vi "Read Configuration Data.vi"(8 "error in":errorcluster) -> (0 "error out":errorcluster, 3 "Configuration Data":T1)   [LabVIEW 2014]
uses:
  Configuration Data.ctl
  controls/MHL Configuration.ctl
  Controller/Controller Configuration.ctl
  Boiler/Boiler Configuration.ctl
  Boiler System Globals.vi
  <vilib>/Utility/config.llb/NI_LVConfig.lvlib
  Controller/Controller.lvlib
  Boiler/Boiler.lvlib
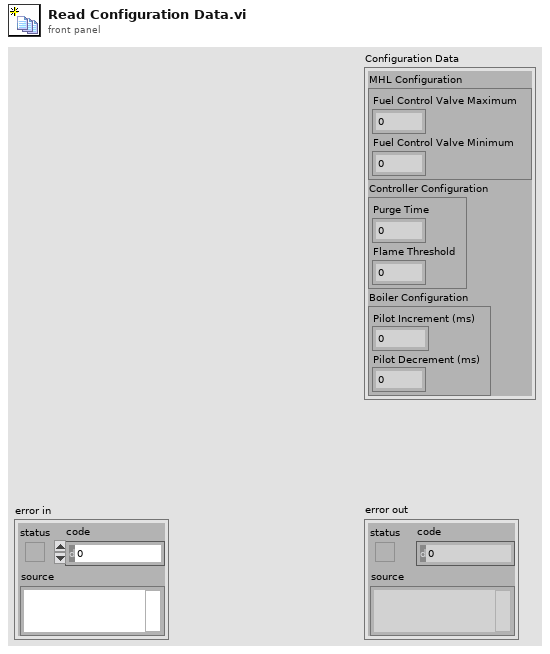
[diagram p1: front panel]
types:
  T1 = typedef "Configuration Data.ctl" = cluster{"MHL Configuration":T2, "Controller Configuration":T3, "Boiler Configuration":T4}
  T2 = typedef "MHL Configuration.ctl" = cluster{"Fuel Control Valve Maximum":dbl, "Fuel Control Valve Minimum":dbl}
  T3 = typedef "Controller.lvlib/Controller Configuration.ctl" = cluster{"Purge Time":u32, "Flame Threshold":u32}
  T4 = typedef "Boiler.lvlib/Boiler Configuration.ctl" = cluster{"Pilot Increment (ms)":u32, "Pilot Decrement (ms)":u32}
  T5 = enum32{"invalid app kind", "Development System", "Run Time System", "Student Edition", "Embedded LabVIEW", "Evaluation", "Custom"}
  T6 = typedef "NI_LVConfig.lvlib/Config Data RefNum.ctl" = refnum<k1>
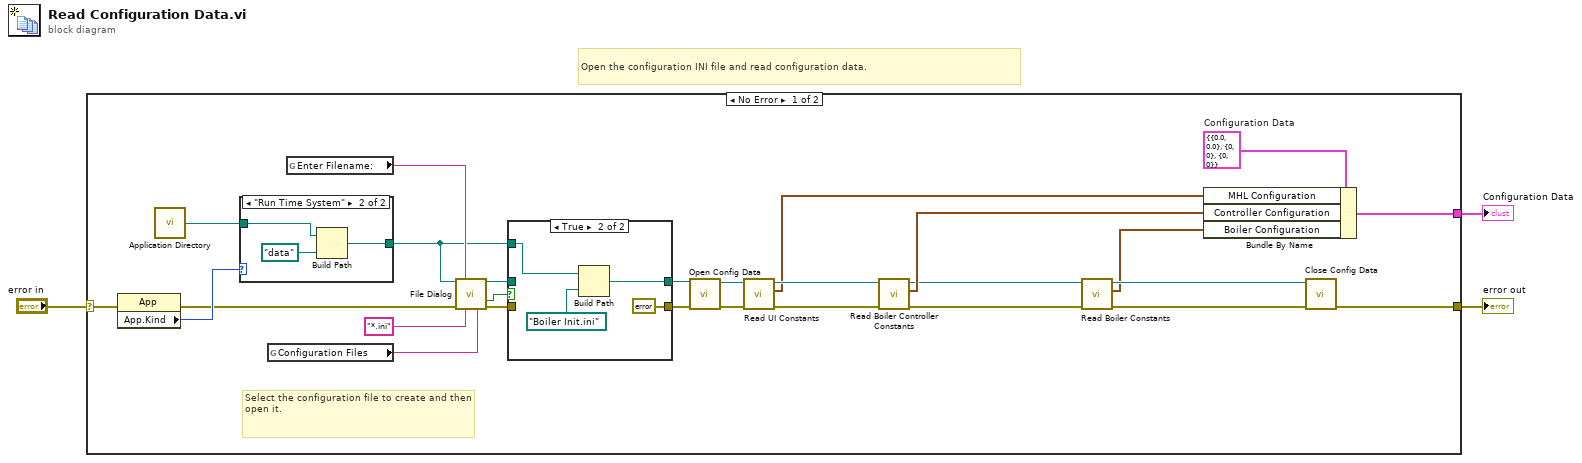
[diagram p0: block diagram]
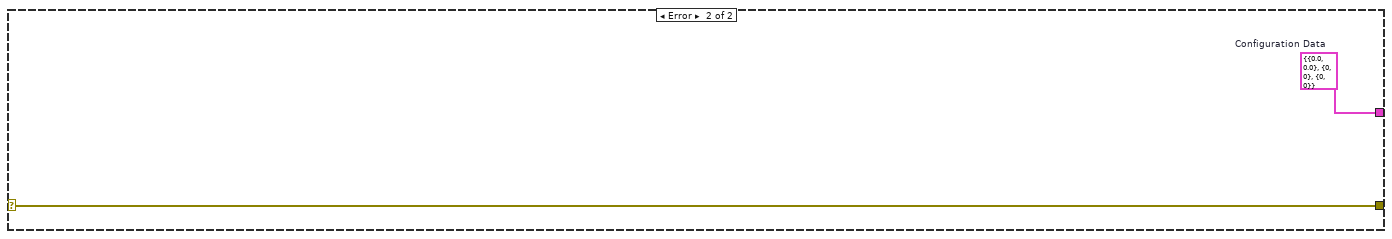
[diagram p4: hidden frame]
diagram:
  # "Open the configuration INI file and read configuration data."
  n1 = case shown="No Error" "error in" {
    selector: "error in" -> [w21 w42]
    tunnel: [w25 w42] -> w3
    tunnel: [w10 w41] -> w1
    frame No Error {
      w12 = T1 {"MHL Configuration"={"Fuel Control Valve Maximum"=0.0, "Fuel Control Valve Minimum"=0.0}, "Controller Configuration"={"Purge Time"=0, "Flame Threshold"=0}, "Boiler Configuration"={"Pilot Increment (ms)"=0, "Pilot Decrement (ms)"=0}}  # Configuration Data
      # "Select the configuration file to create and then open it."
      n2 = property class="App"(error in=w21) -> (error out=w20:errorcluster, "App.Kind"=w23:T5)  [unwired: 1 in, 1 out]
      n3 = call <vilib>:"Application Directory.vi"() -> ("Application Directory"=w22:path)
      n4 = case shown="\"Run Time System\"" w23 {
        tunnel: w22 -> [w37 w40]
        tunnel: [w37 w38] -> w14
        frame Default {
        }
        frame "Run Time System" {
          n5 = Build Path(base path=w40, name or relative path=path "data") -> (appended path=w38:path)
        }
      }
      n6 = global read "Boiler System Globals.vi" "Configuration Files"() -> (w28:string)
      n7 = global read "Boiler System Globals.vi" "Enter Filename:"() -> (w30:string)
      n8 = call "File Dialog"("start path"=w14, "prompt"=w30, "error in"=w20, "pattern (all files)"="*.ini", "pattern label"=w28) -> ("selected path"=w17:path, "cancelled"=w19:bool, "error out"=w18:errorcluster)  [unwired: 7 in, 1 out]
      n9 = case shown="True" w19 {
        tunnel: w18 -> [w32 _]
        tunnel: w17 -> [w31 _]
        tunnel: [w32 errorcluster {"status"=FALSE, "code"=0, "source"=""} ("error out")] -> w16
        tunnel: [w31 w35] -> w15
        tunnel: w14 -> [_ w36]
        frame False {
        }
        frame True {
          n10 = Build Path(base path=w36, name or relative path=path "Boiler Init.ini") -> (appended path=w35:path)
        }
      }
      n11 = call <vilib>:"Open Config Data.vi"("error in (no error)"=w16, "configuration file path"=w15) -> ("error out"=w26:errorcluster, "refnum"=w27:T6)  [unwired: 1 in, 7 out]
      n12 = call "Read UI Constants.vi"("error in"=w26, "CFG File Refnum in"=w27) -> ("error out"=w24:errorcluster, "MHL Configuration"=w11:T2, "CFG File Refnum out"=w13:T6)  [unwired: 7 in]
      n13 = call "Read Boiler Controller Constants.vi"("error in"=w24, "CFG File Refnum in"=w13) -> ("error out"=w7:errorcluster, "Controller Configuration"=w9:T3, "CFG File Refnum out"=w8:T6)  [unwired: 7 in]
      n14 = call "Read Boiler Constants.vi"("error in"=w7, "CFG File Refnum in"=w8) -> ("error out"=w5:errorcluster, "Boiler Configuration"=w4:T4, "CFG File Refnum out"=w6:T6)  [unwired: 7 in]
      n15 = Bundle By Name(cluster=w12, "MHL Configuration"=w11, "Controller Configuration"=w9, "Boiler Configuration"=w4) -> (w10:T1)
      n16 = call <vilib>:"Close Config Data.vi"("error in (no error)"=w5, "refnum"=w6) -> ("error out"=w25:errorcluster)  [unwired: 1 in, 8 out]
    }
    frame Error {
      w41 = T1 {"MHL Configuration"={"Fuel Control Valve Maximum"=0.0, "Fuel Control Valve Minimum"=0.0}, "Controller Configuration"={"Purge Time"=0, "Flame Threshold"=0}, "Boiler Configuration"={"Pilot Increment (ms)"=0, "Pilot Decrement (ms)"=0}}  # Configuration Data
    }
  }
  "error out" <- w3
  "Configuration Data" <- w1
